vi "build compare image.vi"() -> ()   [LabVIEW 2013]
uses:
  <vilib>/picture/picture.llb/imagedata.ctl
panel:
  out "Array 3":dbl[](array[numeric])
  out "Array 2":T1[](array[typedef])
  out "Array":T2(array[cluster])
  out "%'s":dbl[](array[numeric]) format="%.4f"
  out "Possible":i16
  out "Master 2":i32[][](graph)
  out "rect":T3
  out "sum":i16
  out "Intensity":i16[][](graph)
  out "picture":picture
  in  "path to JPEG file":path
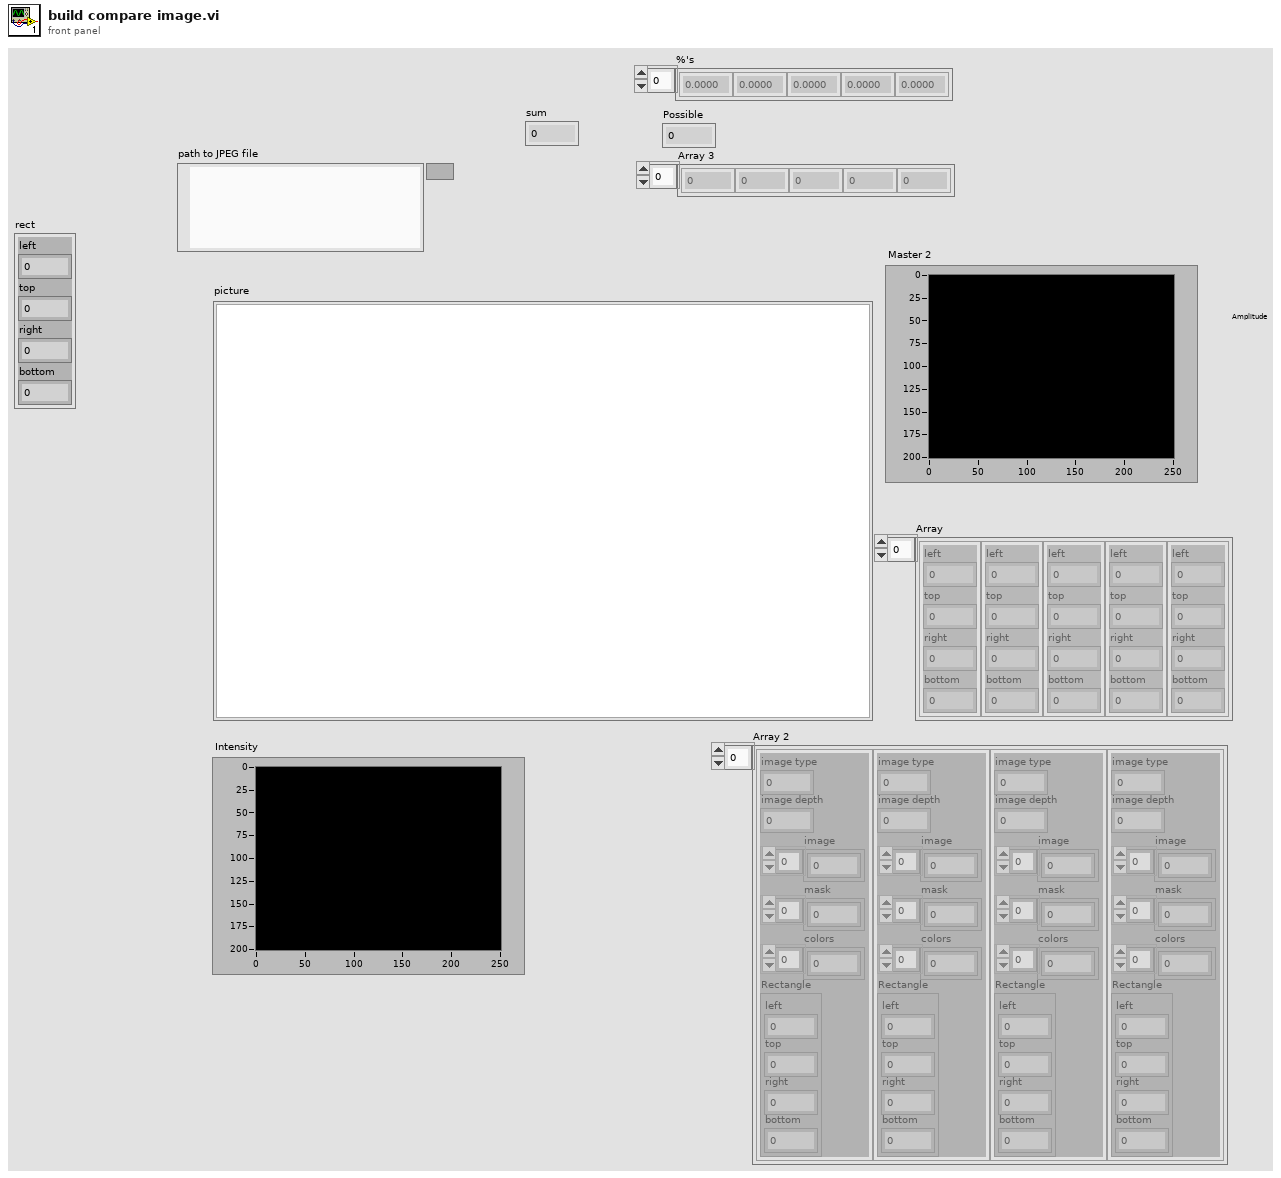
[diagram p1: front panel]
types:
  T1 = typedef "imagedata.ctl" = cluster{"image type":i32, "image depth":i32, "image":u8[], "mask":u8[], "colors":u32[], "Rectangle":cluster{"left":i16, "top":i16, "right":i16, "bottom":i16}}
  T2 = cluster{"left":i16, "top":i16, "right":i16, "bottom":i16}[]
  T3 = cluster{"left":i16, "top":i16, "right":i16, "bottom":i16}
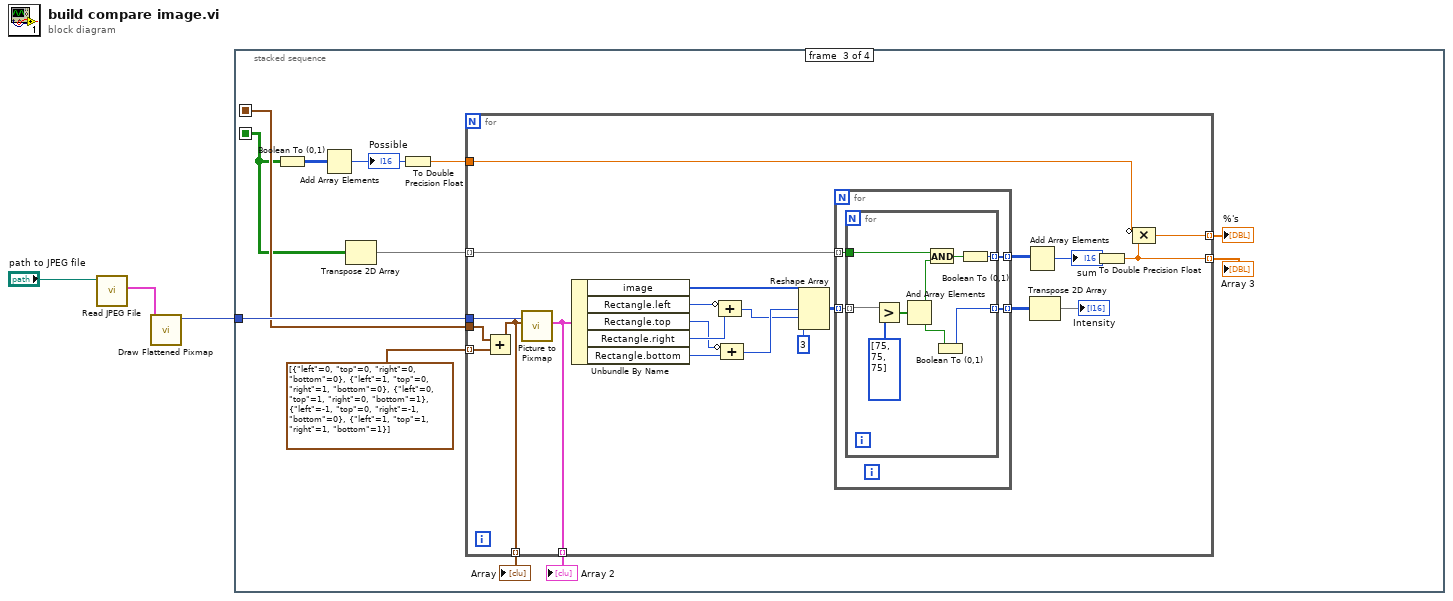
[diagram p0: block diagram]
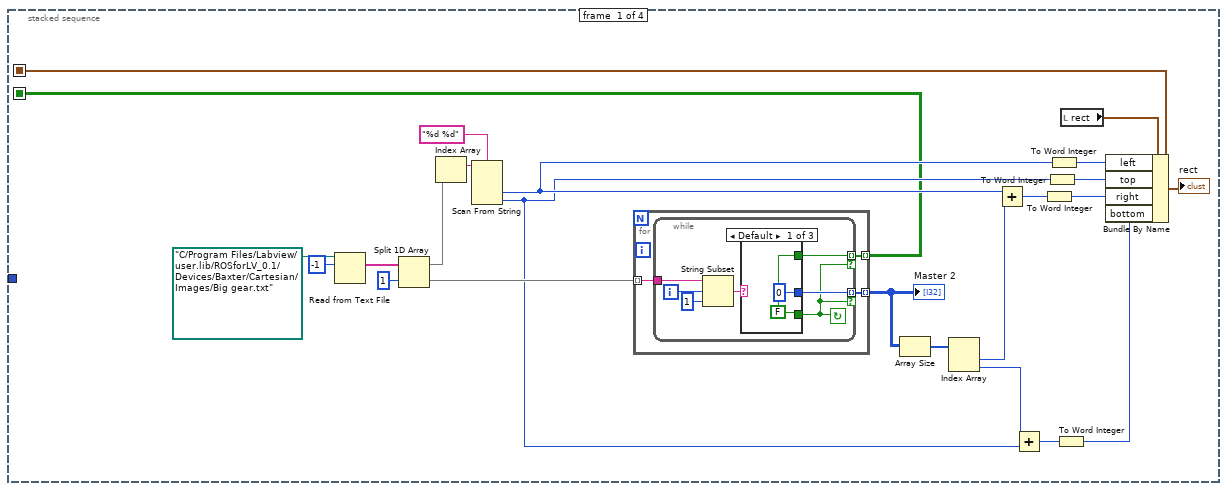
[diagram p2: hidden frame]
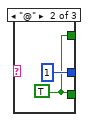
[diagram p3: hidden frame]
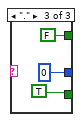
[diagram p4: hidden frame]
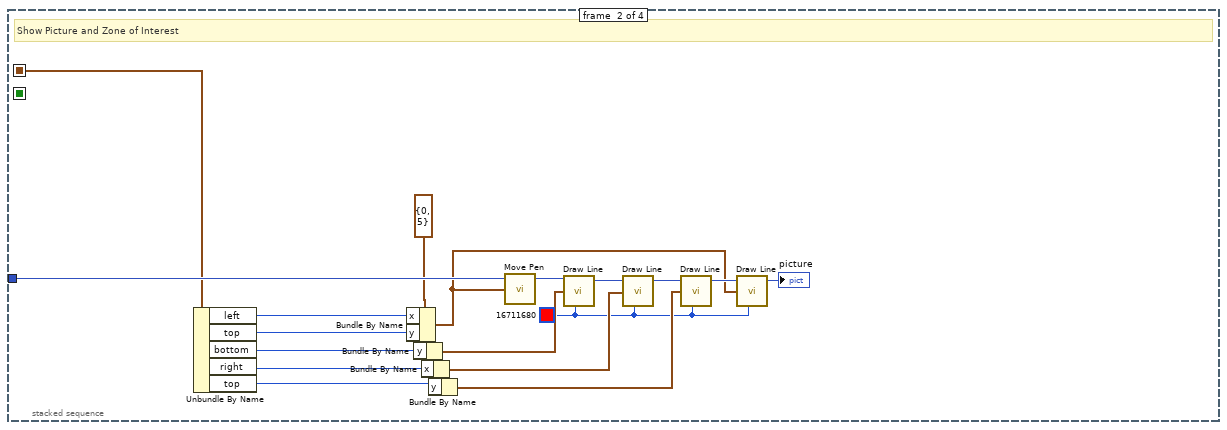
[diagram p5: hidden frame]
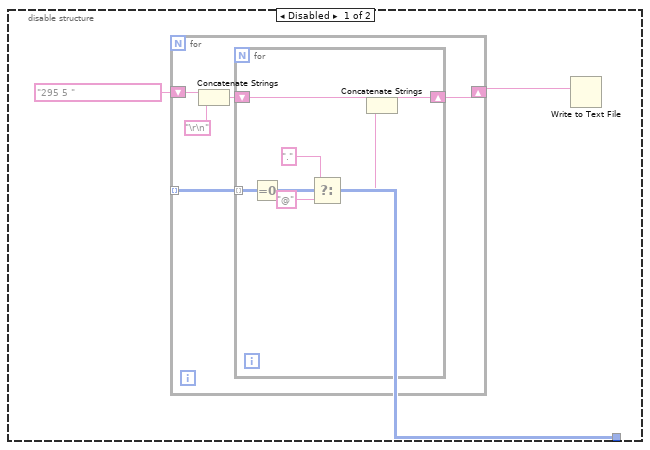
[diagram p7: hidden frame]
diagram:
  n1 = call <vilib>:"Read JPEG File.vi"("path to JPEG file"="path to JPEG file") -> ("image data"=w2:T1)  [unwired: 8 in, 2 out]
  n2 = call <vilib>:"Draw Flattened Pixmap.vi"("image data"=w2) -> ("new picture"=w1:picture)  [unwired: 8 in]
  n3 = stacked-sequence {
    seq-local: [w5 _ _ _] -> [_ w49 w72 _]
    seq-local: [w6 _ _ _] -> [_ _ w69 _]
    tunnel: w1 -> [_ w58 w73 _]
    frame #0 {
      n4 = Read from Text File(file (use dialog)=path "C:/Program Files/Labview/user.lib/ROSforLV_0.1/Devices/Baxter/Cartesian/Images/Big gear.txt", count=-1) -> (text=w18:string[])  [unwired: 2 in, 3 out]
      n5 = Split 1D Array(array=w18, index=1) -> (first subarray=w22:string[], second subarray=w20:string[])
      n6 = Index Array(array=w22) -> (element=w23:string)  [unwired: 1 in]
      n7 = Scan From String(format string="%d %d", input string=w23) -> (output 1=w14:i32, output 2=w13:i32)  [unwired: 4 in, 3 out]
      n8 = for {
        tunnel: [w29] -> w25 mode=indexing
        tunnel: w20 -> [w28] mode=indexing
        tunnel: [w27] -> w6 mode=indexing
        n9 = while {
          tunnel: w28 -> [w34]
          tunnel: [w32] -> w29 mode=indexing if=w30
          tunnel: [w31] -> w27 mode=indexing if=w30
          i -> [w36]
          stop <- w30 continue-if-true
          n10 = String Subset(string=w34, offset (0)=w36, length (rest)=1 ("length (rest)")) -> (substring=w33:string)
          n11 = case shown="Default" w33 {
            tunnel: [w37 w39 TRUE] -> w30
            tunnel: [0 1 0] -> w32
            tunnel: [w37 w39 FALSE] -> w31
            frame Default {
              w37 = FALSE
            }
            frame "@" {
              w39 = TRUE
            }
            frame "." {
            }
          }
        }
      }
      "Master 2" <- w25
      n12 = Array Size(array=w25) -> (size(s)=w26:i32[])
      n13 = Index Array(array=w26) -> (element #1=w16:i32, element #2=w15:i32)  [unwired: 2 in]
      n14 = Add(x=w14, y=w16) -> (x+y=w12:i32)
      n15 = Add(x=w15, y=w13) -> (x+y=w11:i32)
      n16 = To Word Integer(number=w12) -> (16bit integer=w9:i16)
      n17 = To Word Integer(number=w13) -> (16bit integer=w8:i16)
      n18 = To Word Integer(number=w14) -> (16bit integer=w7:i16)
      n19 = To Word Integer(number=w11) -> (16bit integer=w10:i16)
      n20 = local read "rect"() -> (w4:T3)
      n21 = Bundle By Name(cluster=w4, "left"=w7, "top"=w8, "right"=w9, "bottom"=w10) -> (w5:T3)
      "rect" <- w5
    }
    frame #1 {
      w51 = u32 16711680 ("color(black)")
      # "Show Picture and Zone of Interest"
      n22 = Unbundle By Name(w49) -> ("left"=w48:i16, "top"=w47:i16, "bottom"=w46:i16, "right"=w45:i16, "top"=w44:i16)
      n23 = Bundle By Name(cluster=cluster{"x":i16, "y":i16} {"x"=0, "y"=5} ("new position"), "x"=w48, "y"=w47) -> (w50:cluster{"x":i16, "y":i16})
      n24 = Bundle By Name(cluster=w50, "y"=w46) -> (w57:cluster{"x":i16, "y":i16})
      n25 = Bundle By Name(cluster=w57, "x"=w45) -> (w56:cluster{"x":i16, "y":i16})
      n26 = Bundle By Name(cluster=w56, "y"=w44) -> (w55:cluster{"x":i16, "y":i16})
      n27 = call <vilib>:"Move Pen.vi"("new position"=w50, "picture"=w58) -> ("new picture"=w61:picture)  [unwired: 3 in]
      n28 = call <vilib>:"Draw Line.vi"("picture"=w61, "end point"=w57, "color(black)"=w51) -> ("new picture"=w60:picture)  [unwired: 6 in]
      n29 = call <vilib>:"Draw Line.vi"("picture"=w60, "end point"=w56, "color(black)"=w51) -> ("new picture"=w59:picture)  [unwired: 6 in]
      n30 = call <vilib>:"Draw Line.vi"("picture"=w59, "end point"=w55, "color(black)"=w51) -> ("new picture"=w54:picture)  [unwired: 6 in]
      n31 = call <vilib>:"Draw Line.vi"("picture"=w54, "end point"=w50, "color(black)"=w51) -> ("new picture"=→"picture":picture)  [unwired: 6 in]
    }
    frame #2 {
      n32 = Boolean To (0,1)(Boolean=w69) -> (0, 1=w68:i16[][])
      n33 = Add Array Elements(numeric array=w68) -> (sum=w71:i16)
      "Possible" <- w71
      n34 = Transpose 2D Array(2D array=w69) -> (transposed array=w62:bool[][])
      n35 = To Double Precision Float(number=w71) -> (double precision float=w70:dbl)
      n36 = for {
        tunnel: w73 -> [w95]
        tunnel: w72 -> [w77]
        tunnel: [w81] -> w67 mode=indexing
        tunnel: w70 -> [w80]
        tunnel: w62 -> [w79] mode=indexing
        tunnel: T2 [{"left"=0, "top"=0, "right"=0, "bottom"=0}, {"left"=1, "top"=0, "right"=1, "bottom"=0}, {"left"=0, "top"=1, "right"=0, "bottom"=1}, {"left"=-1, "top"=0, "right"=-1, "bottom"=0}, {"left"=1, "top"=1, "right"=1, "bottom"=1}] -> [w78] mode=indexing
        tunnel: [w76] -> w65 mode=indexing
        tunnel: [w75] -> w64 mode=indexing
        tunnel: [w74] -> w63 mode=indexing
        n37 = Add(x=w77, y=w78) -> (x+y=w76:T3)
        n38 = call <vilib>:"Picture to Pixmap.vi"("rect"=w76, "picture"=w95) -> ("image data"=w75:T1)  [unwired: 8 in, 1 out]
        n39 = Unbundle By Name(w75) -> ("image"=w90:u8[], "Rectangle.left"=w94:i16, "Rectangle.top"=w91:i16, "Rectangle.right"=w93:i16, "Rectangle.bottom"=w92:i16)
        n40 = Compound Arithmetic op=ADD(invert w94, w93) -> (w86:i16)
        n41 = Compound Arithmetic op=ADD(invert w91, w92) -> (w87:i16)
        n42 = Reshape Array(w90, w87, w86, 3 ("dimension size")) -> (w88:u8[][][])
        n43 = for {
          tunnel: w88 -> [w99] mode=indexing
          tunnel: [w98] -> w85 mode=indexing
          tunnel: w79 -> [w97] mode=indexing
          tunnel: [w96] -> w83 mode=indexing
          n44 = for {
            tunnel: w99 -> [w107] mode=indexing
            tunnel: [w104] -> w98 mode=indexing
            tunnel: w97 -> [w100]
            tunnel: [w101] -> w96 mode=indexing
            n45 = Greater?(x=w107, y=u8[] [75, 75, 75]) -> (0:w105:bool[])
            n46 = And Array Elements(Boolean array=w105) -> (logical AND=w103:bool)
            n47 = And(x=w100, y=w103) -> (x .and. y?=w102:bool)
            n48 = Boolean To (0,1)(Boolean=w103) -> (0, 1=w104:i16)
            n49 = Boolean To (0,1)(Boolean=w102) -> (0, 1=w101:i16)
          }
        }
        n50 = Add Array Elements(numeric array=w83) -> (sum=w82:i16)
        "sum" <- w82
        n51 = Transpose 2D Array(2D array=w85) -> (transposed array=→"Intensity":i16[][])
        n52 = To Double Precision Float(number=w82) -> (double precision float=w74:dbl)
        n53 = Compound Arithmetic op=MULTIPLY(invert w80, w74) -> (w81:dbl)
      }
      "%'s" <- w67
      "Array" <- w65
      "Array 2" <- w64
      "Array 3" <- w63
    }
    frame #3 {
      n54 = disable-structure shown="Enabled" {
        disable-tunnel: _ -> [w110 _]
        frame Disabled {
          n55 = for {
            tunnel: w110 -> [w115] mode=indexing
            shift-right: [w112] -> w108
            shift-left: "295 5 " -> [w113]
            n56 = Concatenate Strings(w113, "\r\n") -> (w114:string)
            n57 = for {
              tunnel: w115 -> [w122] mode=indexing
              shift-right: [w116] -> w112
              shift-left: w114 -> [w117]
              n58 = Equal To 0?(x=w122) -> (x = 0?=w121:bool)
              n59 = Select(t=".", s=w121, f="@") -> (s? t:f=w118:string)
              n60 = Concatenate Strings(w117, w118) -> (w116:string)
            }
          }
          n61 = Write to Text File(text=w108) -> ()  [unwired: 3 in, 3 out]
        }
        frame Enabled {
        }
      }
    }
  }
